vi "OAT Waterfall Compute Yaxis Offset.vi"(8 "spectral map history":dbl[][](array[numeric]) format="%.2f", 9 "spectral map new":dbl[][](array[numeric]) format="%.2f", 11 "plot settings":T2={"plot color"=0, "grid color"=0, "X shift (rel to total X)"=0.1, "max Z range"=11, "number of spectra"=40} {"max Z range" items=["10^-7", "10^-6", "10^-5", "0.0001", "0.001", "0.01", "0.1", "1", "10", "100", "1000", "auto z range"]; "X shift (rel to total X)" format="%.2f"}) -> (0 "spectral map for display":dbl[][](array[numeric]) format="%.2f", 1 "spectra info":T1, 3 "Y axis offset":i32)   [LabVIEW 2017]
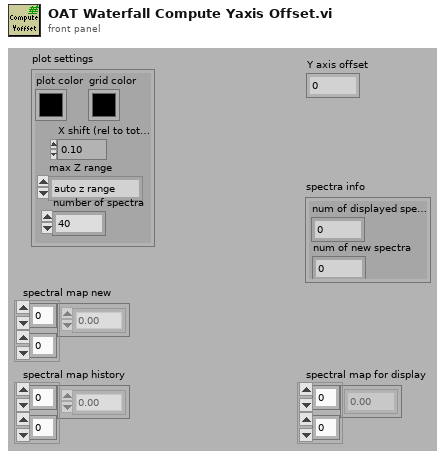
[diagram p1: front panel]
types:
  T1 = cluster{"num of displayed spectra":i32, "num of new spectra":i32}
  T2 = cluster{"plot color":u32, "grid color":u32, "X shift (rel to total X)":dbl, "max Z range":u16, "number of spectra":i32}
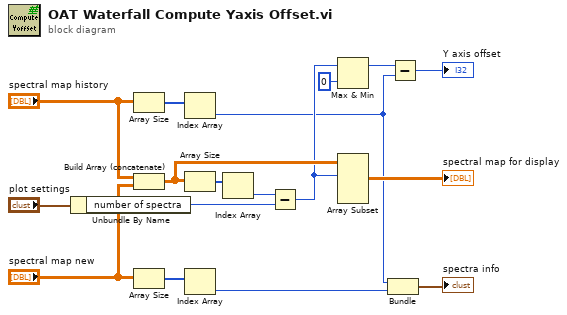
[diagram p0: block diagram]
diagram:
  n1 = Unbundle By Name("plot settings") -> ("number of spectra"=w9:i32)
  n2 = Array Size(array="spectral map history") -> (size(s)=w11:i32[])
  n3 = Build Array (concatenate)("spectral map history", "spectral map new") -> (w14:dbl[][])
  n4 = Array Size(array="spectral map new") -> (size(s)=w12:i32[])
  n5 = Index Array(array=w11) -> (element=w2:i32)  [unwired: 1 in]
  n6 = Array Size(array=w14) -> (size(s)=w17:i32[])
  n7 = Index Array(array=w12) -> (element=w1:i32)  [unwired: 1 in]
  n8 = Index Array(array=w17) -> (element=w4:i32)  [unwired: 1 in]
  n9 = Subtract(x=w4, y=w9) -> (x-y=w8:i32)
  n10 = Max & Min(x=w8, y=0) -> (max(x,y)=w6:i32)  [unwired: 1 out]
  n11 = Array Subset(array=w14, index (row)=w8) -> (→"spectral map for display":dbl[][])  [unwired: 3 in]
  n12 = Bundle(w2, w1) -> (→"spectra info":cluster{i32, i32})  [unwired: 1 in]
  n13 = Subtract(x=w6, y=w2) -> (x-y=→"Y axis offset":i32)
